vi "fpga_2CHInputValid.vi"(3 "input data valid":bool, 5 "Channel number":u8) -> (0 "input valid":bool, 1 "1CH?":bool, 2 "Channel number":u8)   [LabVIEW 2011, in "NI_EP_Resample_FPGA.lvlib"]
uses:
  <vilib>/addons/Electrical Power/PQ/Resampling/NI_EP_Resample_FPGA.lvlib
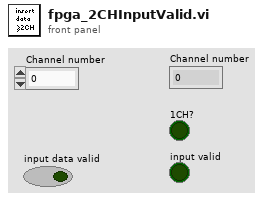
[diagram p1: front panel]
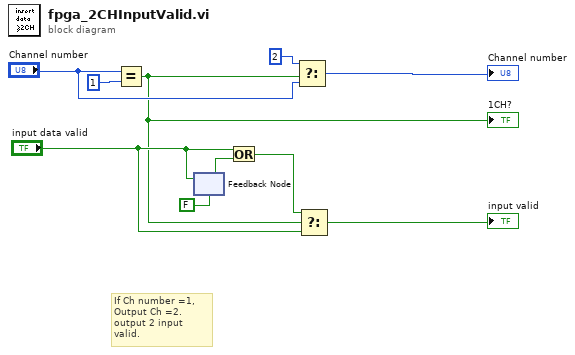
[diagram p0: block diagram]
diagram:
  # "If Ch number =1,\nOutput Ch =2.\noutput 2 input valid."
  n1 = Equal?(x="Channel number", y=u8 1) -> (x = y?=w1:bool)
  "1CH?" <- w1
  n2 = feedback-in #1("input data valid") -> ()
  n3 = feedback #1(FALSE ("input data valid")) -> (w5:bool)
  n4 = Or(x="input data valid", y=w5) -> (x .or. y?=w4:bool)
  n5 = Select(t=u8 2 ("y"), s=w1, f="Channel number") -> (s? t:f=→"Channel number":u8)
  n6 = Select(t=w4, s=w1, f="input data valid") -> (s? t:f=→"input valid":bool)
